vi "Get Averaging Period.vi"(8 "error in (no error)":errorcluster, 11 "EPU452 in":refnum<class "EPU452.lvclass">) -> (0 "error out":errorcluster, 1 "Period":dbl, 2 "Response":string, 3 "EPU452 out":refnum<class "EPU452.lvclass">)   [LabVIEW 2018, in "EPU452.lvclass"]
uses:
  EPU452.lvclass
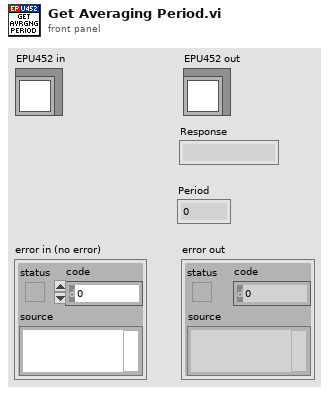
[diagram p1: front panel]
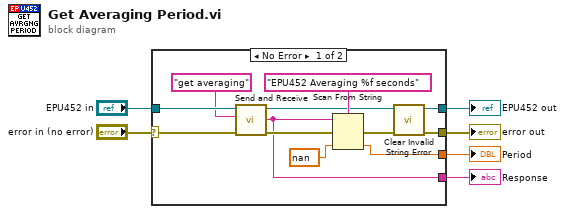
[diagram p0: block diagram]
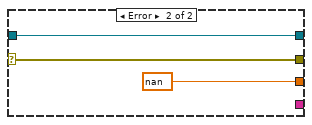
[diagram p2: hidden frame]
diagram:
  n1 = case shown="No Error" "error in (no error)" {
    selector: "error in (no error)" -> [w17 w21]
    tunnel: [w10 w21] -> w5
    tunnel: [w9 w20] -> w3
    tunnel: "EPU452 in" -> [w18 w20]
    tunnel: [w8 nan ("default value 1")] -> w2
    tunnel: [w7 _] -> w1
    frame No Error {
      n2 = call "Send and Receive.vi"("error in (no error)"=w17, "Command"="get averaging", "EPU452 in"=w18) -> ("error out"=w13:errorcluster, "Response"=w7:string, "EPU452 out"=w11:refnum<class "EPU452.lvclass">)  [unwired: 6 in]
      n3 = Scan From String(format string="EPU452 Averaging %f seconds" ("Command"), input string=w7, error in=w13, default 1=nan ("default value 1")) -> (error out=w12:errorcluster, output 1=w8:dbl)  [unwired: 1 in, 2 out]
      n4 = call "Clear Invalid String Error.vi"("error in (no error)"=w12, "EPU452 in"=w11) -> ("error out"=w10:errorcluster, "EPU452 out"=w9:refnum<class "EPU452.lvclass">)  [unwired: 8 in]
    }
    frame Error {
    }
  }
  "error out" <- w5
  "EPU452 out" <- w3
  "Period" <- w2
  "Response" <- w1
